vi "Result.Parse STD OUT Text, Create Result Data.vi"(4 "UUTDir":path, 6 "Prefix":string, 7 "Category":string, 8 "Version Name":string, 9 "Error Code":i32, 10 "Task Name":string, 11 "StdOut":string) -> (0 "Error":errorcluster, 1 "SW Ver":T4[](array[typedef]), 3 "Meas":T2[](array[typedef]) {"Status" items=["LOG", "PASS", "FAIL", "ERROR"]}, 5 "Data Files":T1[](array[typedef]))   [LabVIEW 2024]
uses:
  Result XML/TestResult.SW Item.ctl
  Result.Measurement Item.ctl
  Result.Measurement and Attribute Item Status.ctl
  Reports/Report.Result FileDataObject.ctl
  Errors/Error.Error Code List.ctl
  <vilib>/Utility/error.llb/Trim Whitespace One-Sided.vi
  <vilib>/KATE/Files/File Utils.lvlib
  Errors.lvlib
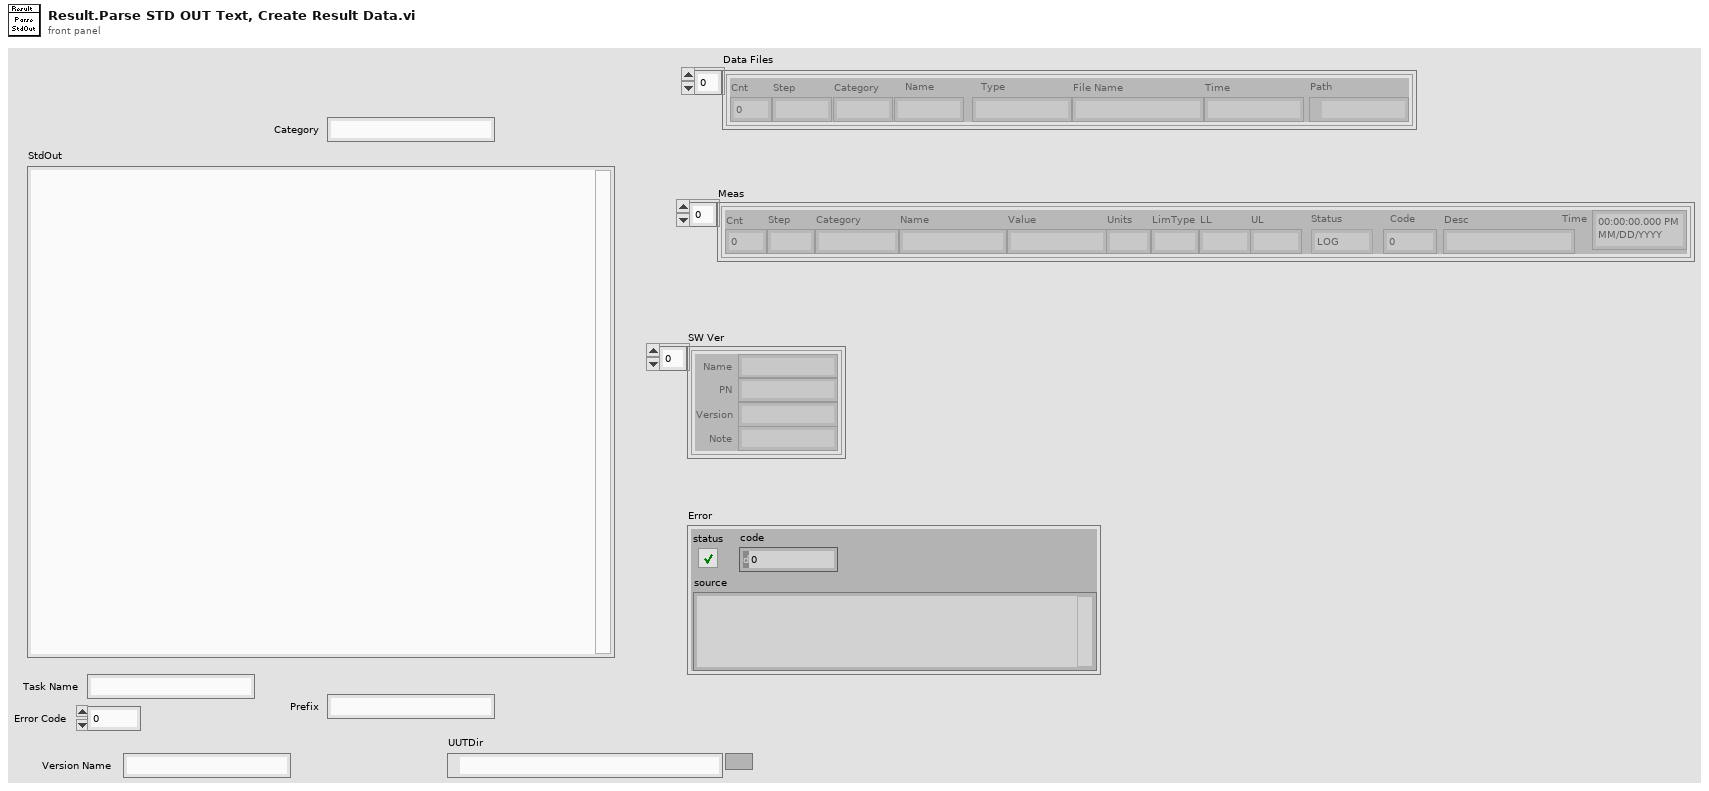
[diagram p1: front panel]
types:
  T1 = typedef "Report.Result FileDataObject.ctl" = cluster{"Cnt":i32, "Step":string, "Category":string, "Name":string, "Type":string, "File Name":string, "Time":string, "Path":path}
  T2 = typedef "Result.Measurement Item.ctl" = cluster{"Cnt":i32, "Step":string, "Category":string, "Name":string, "Value":string, "Units":string, "LimType":string, "LL":string, "UL":string, "Status":T3, "Code":i32, "Desc":string, "Time":timestamp}
  T3 = typedef "Result.Measurement and Attribute Item Status.ctl" = i32
  T4 = typedef "TestResult.SW Item.ctl" = cluster{"Name":string, "PN":string, "Version":string, "Note":string}
  T5 = cluster{"Meas":T2[], "SW Ver":T4[], "Error":errorcluster, "Data Files":T1[]}
  T6 = typedef "EQMF.lvlib/Errors.lvlib/Error.Error Code List.ctl" = i32
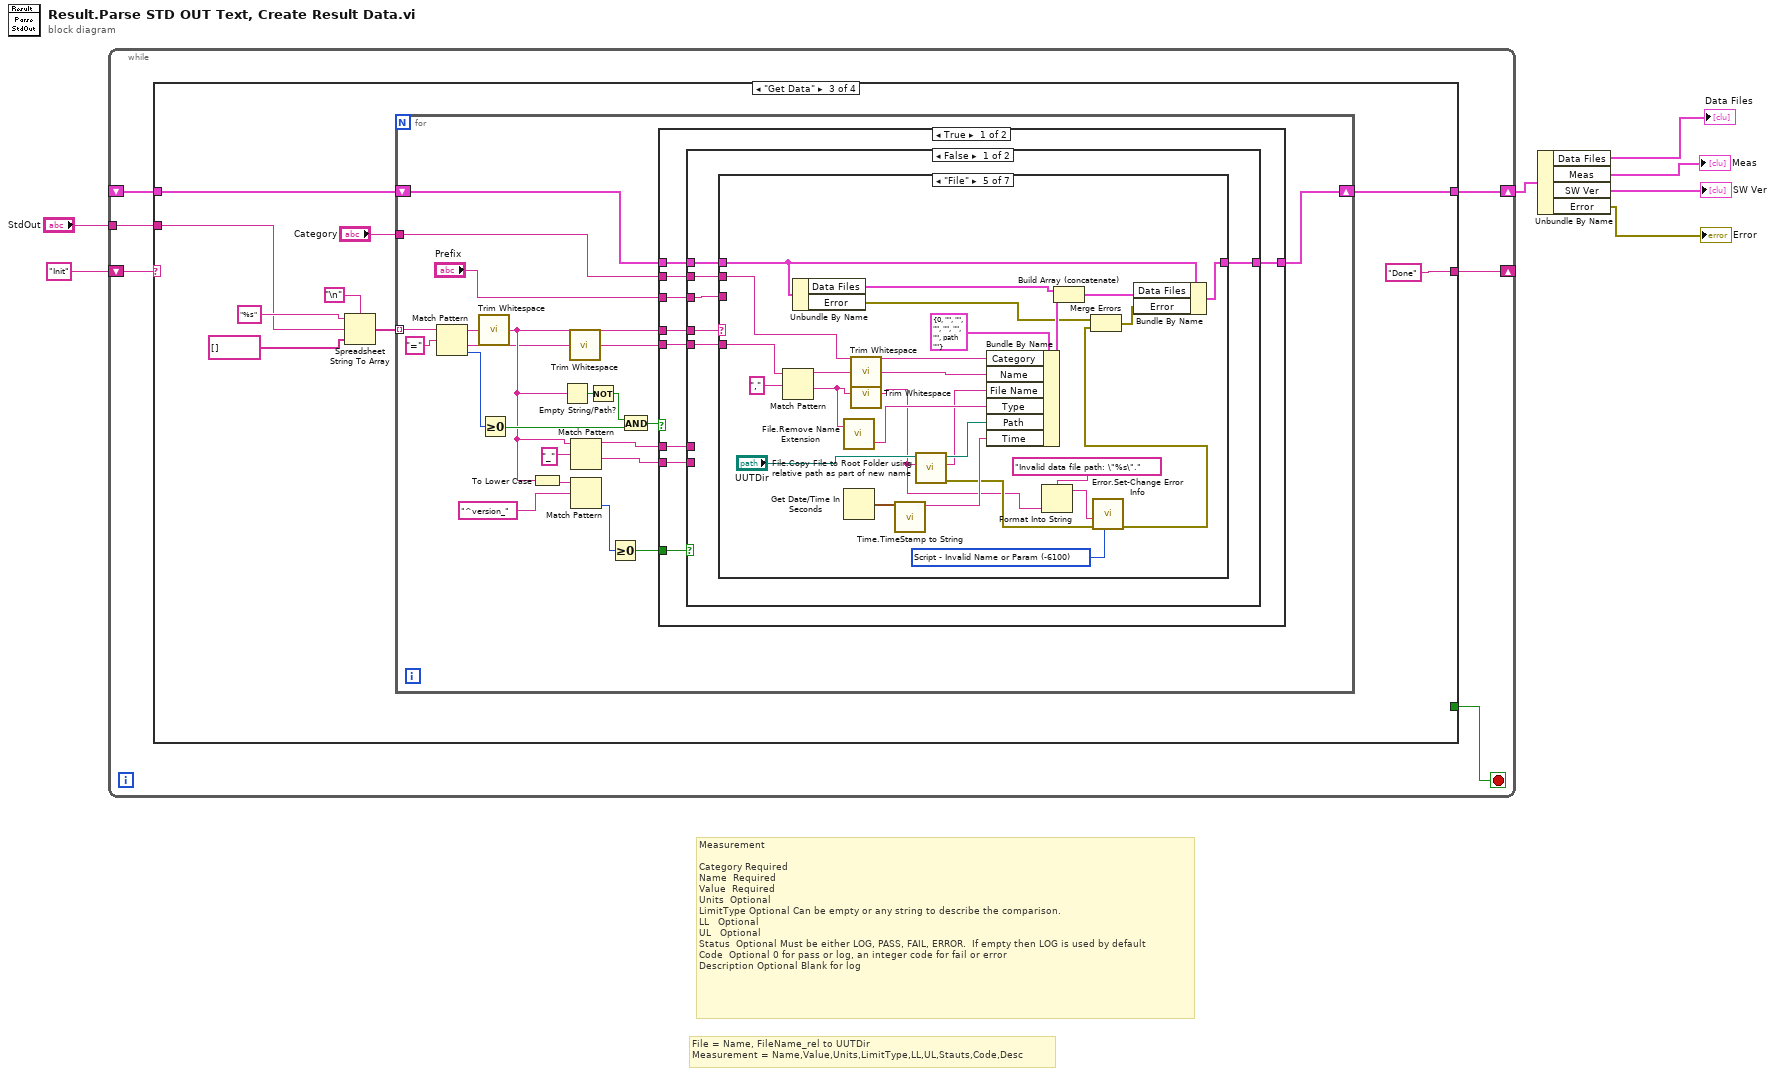
[diagram p0: block diagram]
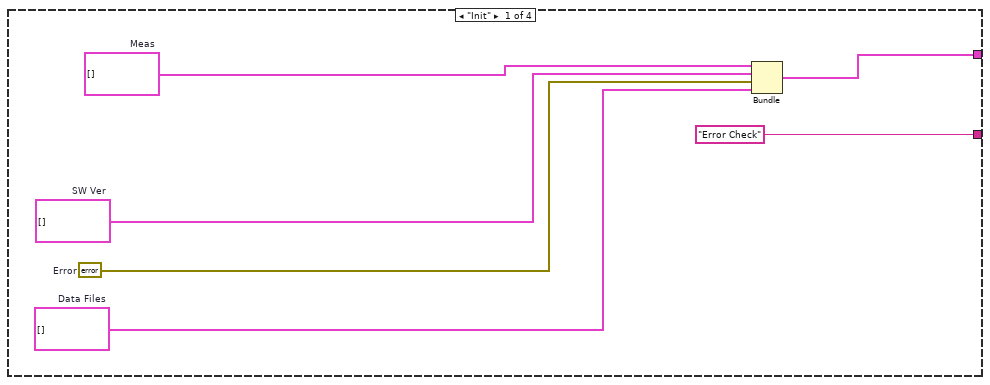
[diagram p2: hidden frame]
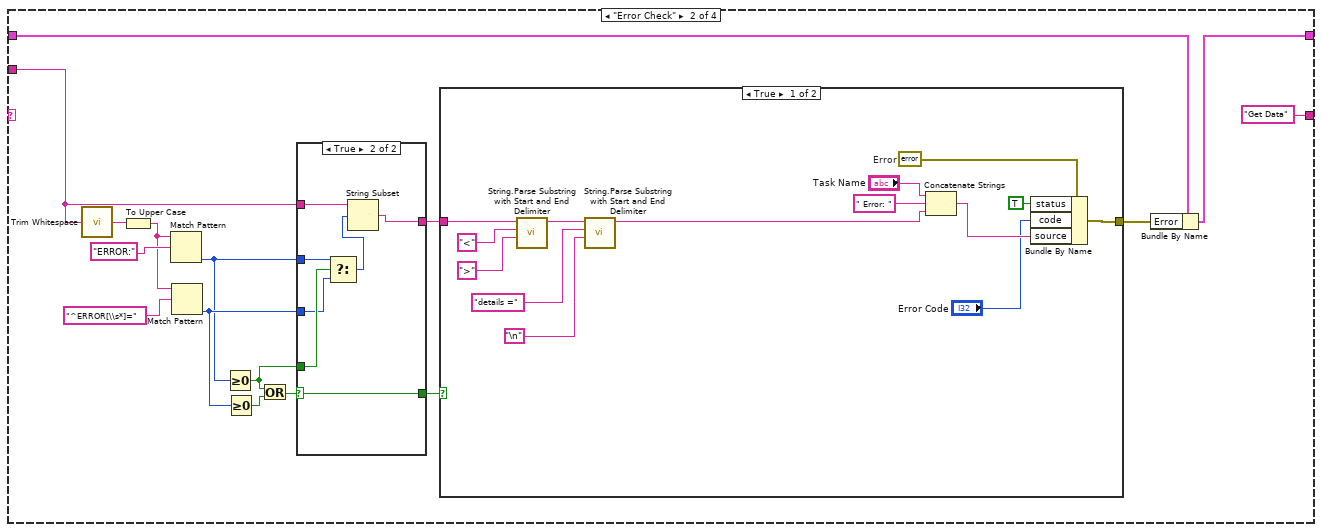
[diagram p3: hidden frame]
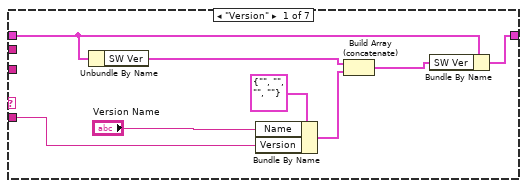
[diagram p6: hidden frame]
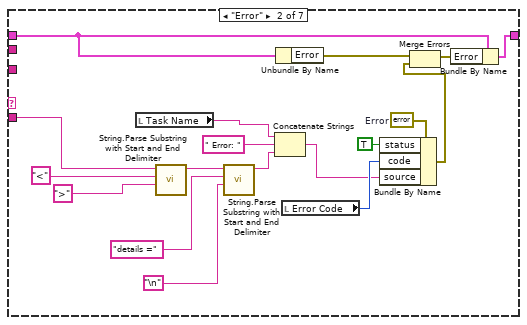
[diagram p7: hidden frame]
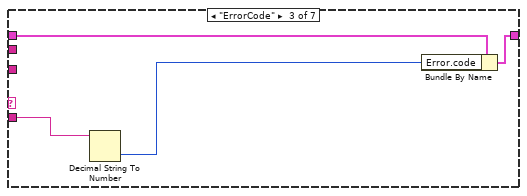
[diagram p8: hidden frame]
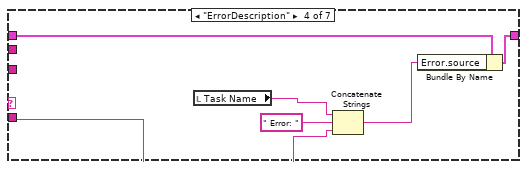
[diagram p9: hidden frame]
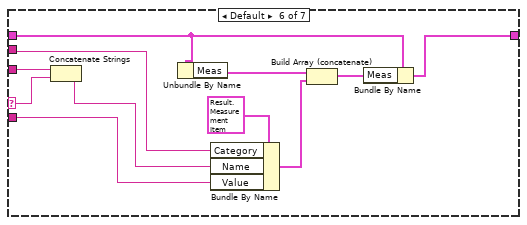
[diagram p10: hidden frame]
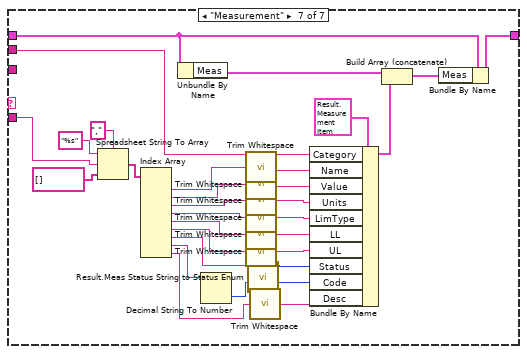
[diagram p11: hidden frame]
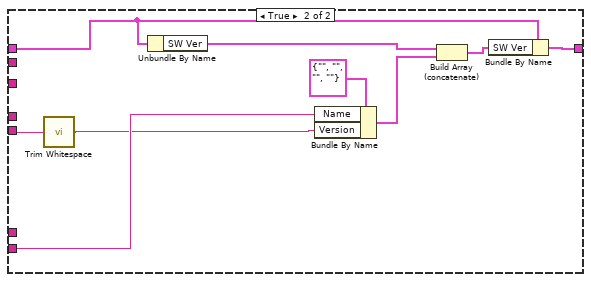
[diagram p12: hidden frame]
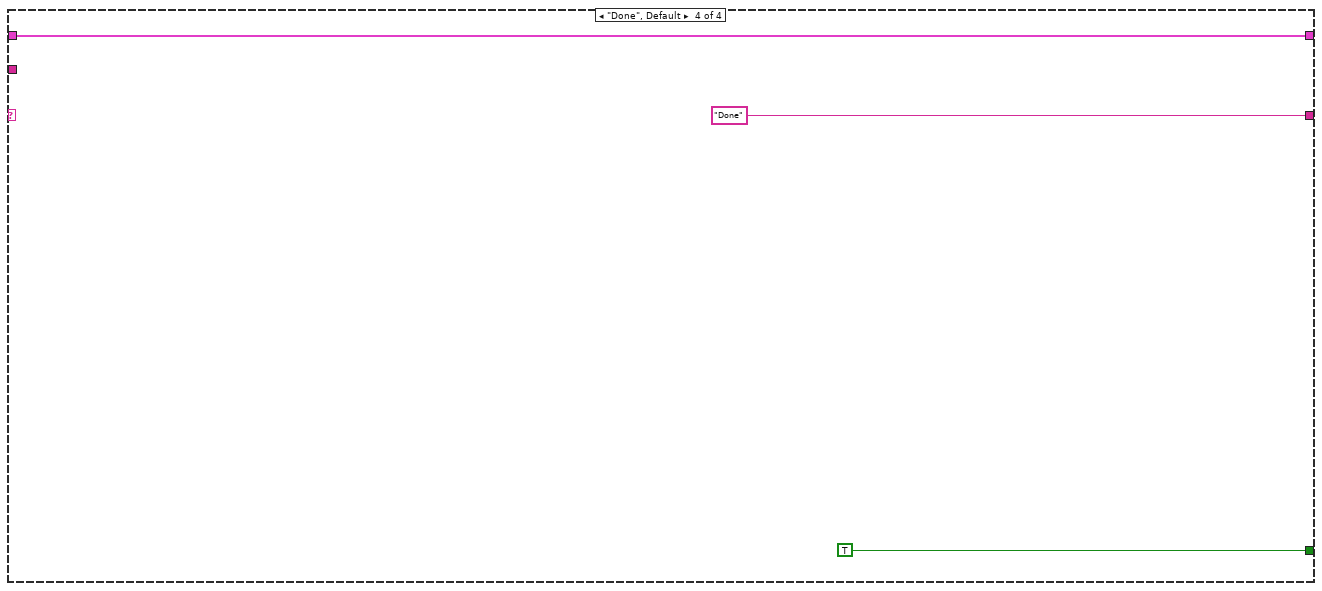
[diagram p14: hidden frame]
diagram:
  # "File = Name, FileName_rel to UUTDir\nMeasurement = Name,Value,Units,LimitType,LL,UL,Stauts,Code,Desc"
  # "Measurement\n\nCategory\tRequired\nName\t\tRequired\nValue\t\tRequired\nUnits\t\tOptional\t\nLimitType\tOptional\tCan be empty or any string to describe the comparison. \nLL \t\tOptional\nUL \t\tOptional\nStatus\t\tOptional\tMust be either LOG, PASS, FAIL, ERROR.  If empty then LOG is used by default\nCode\t\tOptional\t0 for pass or log, an integer code for fail or error\nDescription\tOptional\tBlank for log"
  n1 = while {
    tunnel: "StdOut" -> [w13]
    shift-right: [w9] -> _
    shift-left: "Init" -> [w12]
    shift-right: [w10] -> w5
    shift-left: _ -> [w11]
    stop <- w8 stop-if-true
    n2 = case shown="\"Get Data\"" w12 {
      tunnel: w13 -> [_ w20 w63 _]
      tunnel: w11 -> [_ w34 w60 w217]
      tunnel: [w17 w33 w58 w217] -> w10
      tunnel: ["Error Check" "Get Data" "Done" "Done"] -> w9
      tunnel: [_ _ _ TRUE] -> w8
      frame "Init" {
        w14 = T1[] []  # Data Files
        w15 = errorcluster {"status"=FALSE, "code"=0, "source"=""}  # Error
        w19 = T2[] []  # Meas
        w18 = T4[] []  # SW Ver
        n3 = Bundle("Meas"=w19, "SW Ver"=w18, "Error"=w15, "Data Files"=w14) -> (w17:T5)  [unwired: 1 in]
      }
      frame "Error Check" {
        n4 = call <vilib>:"Trim Whitespace.vi"("string"=w20) -> ("trimmed string"=w21:string)  [unwired: 1 in]
        n5 = To Upper Case(1:w21) -> (0:w29:string)
        n6 = Match Pattern(string=w29, regular expression="ERROR:") -> (offset past match=w25:i32)  [unwired: 1 in, 3 out]
        n7 = Match Pattern(string=w29, regular expression="^ERROR[\\s*]=") -> (offset past match=w26:i32)  [unwired: 1 in, 3 out]
        n8 = Greater Or Equal To 0?(x=w25) -> (x >= 0?=w24:bool)
        n9 = Greater Or Equal To 0?(x=w26) -> (x >= 0?=w28:bool)
        n10 = Or(x=w24, y=w28) -> (x .or. y?=w27:bool)
        n11 = case shown="True" w27 {
          selector: w27 -> [w36 w37]
          tunnel: w26 -> [_ w40]
          tunnel: w25 -> [_ w42]
          tunnel: w20 -> [_ w43]
          tunnel: w24 -> [_ w41]
          tunnel: [_ w38] -> w23
          tunnel: [w36 w37] -> w22
          frame False {
          }
          frame True {
            n12 = Select(t=w42, s=w41, f=w40) -> (s? t:f=w39:i32)
            n13 = String Subset(string=w43, offset (0)=w39) -> (substring=w38:string)  [unwired: 1 in]
          }
        }
        n14 = case shown="True" w22 {
          tunnel: w23 -> [w50 _]
          tunnel: [w51 _] -> w31
          frame True {
            w57 = errorcluster {"status"=FALSE, "code"=0, "source"=""}  # Error
            n15 = call "String.Parse Substring with Start and End Delimiter.vi"("Delimiter2"=">", "Delimiter1"="<", "String In"=w50) -> ("String Out"=w47:string)  [unwired: 7 in, 1 out]
            n16 = call "String.Parse Substring with Start and End Delimiter.vi"("Delimiter2"="\n", "Delimiter1"="details =", "String In"=w47) -> ("String Out"=w44:string)  [unwired: 7 in, 1 out]
            n17 = Concatenate Strings("Task Name", " Error: ", w44) -> (w53:string)
            n18 = Bundle By Name(cluster=w57, "status"=TRUE, "code"="Error Code", "source"=w53) -> (w51:errorcluster)
          }
          frame False {
          }
        }
        n19 = Bundle By Name(cluster=w34, "Error"=w31) -> (w33:T5)
      }
      frame "Get Data" {
        n20 = Spreadsheet String To Array(delimiter (Tab)="\n", format string="%s" ("spreadsheet string"), spreadsheet string=w63, array type (2D Dbl)=string[] []) -> (array=w61:string[])
        n21 = for {
          tunnel: w61 -> [w88] mode=indexing
          shift-right: [w85] -> w58
          shift-left: w60 -> [w86]
          tunnel: "Category" -> [w78]
          n22 = Match Pattern(string=w88, regular expression="=") -> (before substring=w84:string, after substring=w68:string, offset past match=w83:i32)  [unwired: 1 in, 1 out]
          n23 = call <vilib>:"Trim Whitespace.vi"("string"=w84) -> ("trimmed string"=w69:string)  [unwired: 1 in]
          n24 = Greater Or Equal To 0?(x=w83) -> (x >= 0?=w80:bool)
          n25 = To Lower Case(string=w69) -> (all lower case string=w73:string)
          n26 = Empty String/Path?(string/path=w69) -> (empty?=w82:bool)
          n27 = call <vilib>:"Trim Whitespace.vi"("string"=w68) -> ("trimmed string"=w67:string)  [unwired: 1 in]
          n28 = Match Pattern(string=w69, regular expression="_") -> (before substring=w72:string, after substring=w71:string)  [unwired: 1 in, 2 out]
          n29 = Match Pattern(string=w73, regular expression="^version_") -> (offset past match=w76:i32)  [unwired: 1 in, 3 out]
          n30 = Not(x=w82) -> (.not. x?=w81:bool)
          n31 = Greater Or Equal To 0?(x=w76) -> (x >= 0?=w75:bool)
          n32 = And(x=w81, y=w80) -> (x .and. y?=w79:bool)
          n33 = case shown="True" w79 {
            tunnel: w86 -> [w95 w216]
            tunnel: [w94 w216] -> w85
            tunnel: w67 -> [w97 _]
            tunnel: w69 -> [w93 _]
            tunnel: w78 -> [w96 _]
            tunnel: "Prefix" -> [w92 _]
            tunnel: w72 -> [w89 _]
            tunnel: w71 -> [w90 _]
            tunnel: w75 -> [w91 _]
            frame True {
              n34 = case shown="False" w91 {
                tunnel: w97 -> [w103 w208]
                tunnel: w96 -> [w102 _]
                tunnel: w95 -> [w101 w210]
                tunnel: [w100 w211] -> w94
                tunnel: w93 -> [w99 _]
                tunnel: w92 -> [w98 _]
                tunnel: w90 -> [_ w209]
                tunnel: w89 -> [_ _]
                frame False {
                  n35 = case shown="\"File\"" w99 {
                    selector: w99 -> [_ _ _ _ _ w171 _]
                    tunnel: w103 -> [w104 w112 w130 w135 w152 w176 w196]
                    tunnel: w102 -> [_ _ _ _ w159 w172 w204]
                    tunnel: w101 -> [w110 w128 w133 w139 w148 w175 w206]
                    tunnel: [w109 w129 w132 w138 w165 w174 w205] -> w100
                    tunnel: w98 -> [_ _ _ _ _ w173 _]
                    frame "Version" {
                      n36 = Unbundle By Name(w110) -> ("SW Ver"=w107:T4[])
                      n37 = Bundle By Name(cluster=T4 {"Name"="", "PN"="", "Version"="", "Note"=""} ("SW_Item"), "Name"="Version Name", "Version"=w104) -> (w106:T4)
                      n38 = Build Array (concatenate)(w107, w106) -> (w108:T4[])
                      n39 = Bundle By Name(cluster=w110, "SW Ver"=w108) -> (w109:T5)
                    }
                    frame "Error" {
                      w115 = errorcluster {"status"=FALSE, "code"=0, "source"=""}  # Error
                      n40 = local read "Task Name"() -> (w124:string)
                      n41 = call "String.Parse Substring with Start and End Delimiter.vi"("Delimiter2"=">", "Delimiter1"="<", "String In"=w112) -> ("String Out"=w122:string)  [unwired: 7 in, 1 out]
                      n42 = call "String.Parse Substring with Start and End Delimiter.vi"("Delimiter2"="\n", "Delimiter1"="details =", "String In"=w122) -> ("String Out"=w123:string)  [unwired: 7 in, 1 out]
                      n43 = Concatenate Strings(w124, " Error: ", w123) -> (w121:string)
                      n44 = Unbundle By Name(w128) -> ("Error"=w126:errorcluster)
                      n45 = local read "Error Code"() -> (w125:i32)
                      n46 = Bundle By Name(cluster=w115, "status"=TRUE, "code"=w125, "source"=w121) -> (w113:errorcluster)
                      n47 = Merge Errors(w126, w113) -> (w127:errorcluster)
                      n48 = Bundle By Name(cluster=w128, "Error"=w127) -> (w129:T5)
                    }
                    frame "ErrorCode" {
                      n49 = Decimal String To Number(string=w130) -> (number=w131:i32)  [unwired: 2 in, 1 out]
                      n50 = Bundle By Name(cluster=w133, "Error.code"=w131) -> (w132:T5)
                    }
                    frame "ErrorDescription" {
                      n51 = local read "Task Name"() -> (w137:string)
                      n52 = Concatenate Strings(w137, " Error: ", w135) -> (w134:string)
                      n53 = Bundle By Name(cluster=w139, "Error.source"=w134) -> (w138:T5)
                    }
                    frame "File" {
                      w144 = T6 -6100 items=["No Error"=0, "Abort"=-2, "Misc"=-5000, "Fixture Error"=-5100, "File IO - General"=-5200, "FIle IO - Config Error"=-5201, "Instrument - General"=-5300, "Instrument - Serial Com"=-5301, "Instrument - Camera"=-5302, "Instrument - PS"=-5303, "Instrument - Oscilloscope"=-5304, "Instrument - Function Gen"=-5305, "Instrument - Load"=-5306, "Instrument - Meter"=-5307, "Instrument - Power Control"=-5308, "Instrument - Motion"=-5309, "Instrument - RF"=-5310, "System Exe"=-5400, "Image Processing"=-5500, "Communication"=-5600, "Script - Syntax Error"=-6000, "Script - Invalid Name or Param"=-6100, "Script - Timeout"=-6200, "Invalid Data"=-6300, "FW Update Error"=-6500] ("Std Code")
                      n54 = Match Pattern(string=w152, regular expression=",") -> (before substring=w157:string, after substring=w155:string)  [unwired: 1 in, 2 out]
                      n55 = Unbundle By Name(w148) -> ("Data Files"=w163:T1[], "Error"=w146:errorcluster)
                      n56 = call <vilib>:"File.Remove Name Extension.vi"("File Name"=w155) -> ("Ext"=w156:string)  [unwired: 1 in, 1 out]
                      n57 = Get Date/Time In Seconds() -> (seconds since 1Jan1904=w154:timestamp)
                      n58 = call <vilib>:"Trim Whitespace.vi"("string"=w157) -> ("trimmed string"=w158:string)  [unwired: 1 in]
                      n59 = call <vilib>:"Trim Whitespace.vi"("string"=w155) -> ("trimmed string"=w141:string)  [unwired: 1 in]
                      n60 = call "Time.TimeStamp to String.vi"("Time Stamp in"=w154) -> ("Time String Out"=w153:string)  [unwired: 10 in]
                      n61 = call "File.Copy File to Root Folder using relative path as part of new name.vi"("Relative Path"=w141, "Root Path"="UUTDir") -> ("error out"=w145:errorcluster, "New File Name"=w149:string, "Adjusted Path"=w150:path)  [unwired: 6 in, 1 out]
                      n62 = Bundle By Name(cluster=T1 {"Cnt"=0, "Step"="", "Category"="", "Name"="", "Type"="", "File Name"="", "Time"="", "Path"=path ""} ("FileData Object"), "Category"=w159, "Name"=w158, "File Name"=w149, "Type"=w156, "Path"=w150, "Time"=w153) -> (w162:T1)
                      n63 = Format Into String(format string="Invalid data file path: \"%s\".", w141) -> (resulting string=w142:string)  [unwired: 2 in, 1 out]
                      n64 = Build Array (concatenate)(w163, w162) -> (w164:T1[])
                      n65 = call "Error.Set-Change Error Info.vi"("Std Code"=w144, "error in"=w145, "Description"=w142) -> ("error out"=w140:errorcluster)  [unwired: 8 in]
                      n66 = Merge Errors(w146, w140) -> (w147:errorcluster)
                      n67 = Bundle By Name(cluster=w148, "Data Files"=w164, "Error"=w147) -> (w165:T5)
                    }
                    frame Default {
                      n68 = Concatenate Strings(w173, w171) -> (w170:string)
                      n69 = Unbundle By Name(w175) -> ("Meas"=w168:T2[])
                      n70 = Bundle By Name(cluster=T2 {"Cnt"=0, "Step"="", "Category"="", "Name"="", "Value"="", "Units"="", "LimType"="", "LL"="", "UL"="", "Status"=0, "Code"=0, "Desc"="", "Time"=timestamp(0 s since 1904-01-01)} ("Meas"), "Category"=w172, "Name"=w170, "Value"=w176) -> (w167:T2)
                      n71 = Build Array (concatenate)(w168, w167) -> (w166:T2[])
                      n72 = Bundle By Name(cluster=w175, "Meas"=w166) -> (w174:T5)
                    }
                    frame "Measurement" {
                      n73 = Spreadsheet String To Array(delimiter (Tab)="," ("spreadsheet string"), format string="%s" ("spreadsheet string"), spreadsheet string=w196, array type (2D Dbl)=string[] []) -> (array=w195:string[])
                      n74 = Index Array(array=w195) -> (element #1=w194:string, element #2=w193:string, element #3=w190:string, element #4=w189:string, element #5=w188:string, element #6=w187:string, element #7=w180:string, element #8=w179:string, element #9=w177:string)  [unwired: 9 in]
                      n75 = Unbundle By Name(w206) -> ("Meas"=w202:T2[])
                      n76 = Decimal String To Number(string=w179) -> (number=w178:i32)  [unwired: 2 in, 1 out]
                      n77 = call <vilib>:"Trim Whitespace.vi"("string"=w194) -> ("trimmed string"=w192:string)  [unwired: 1 in]
                      n78 = call <vilib>:"Trim Whitespace.vi"("string"=w193) -> ("trimmed string"=w191:string)  [unwired: 1 in]
                      n79 = call <vilib>:"Trim Whitespace.vi"("string"=w190) -> ("trimmed string"=w186:string)  [unwired: 1 in]
                      n80 = call <vilib>:"Trim Whitespace.vi"("string"=w189) -> ("trimmed string"=w185:string)  [unwired: 1 in]
                      n81 = call <vilib>:"Trim Whitespace.vi"("string"=w188) -> ("trimmed string"=w182:string)  [unwired: 1 in]
                      n82 = call <vilib>:"Trim Whitespace.vi"("string"=w187) -> ("trimmed string"=w184:string)  [unwired: 1 in]
                      n83 = call "Result.Meas Status String to Status Enum.vi"("Status Str"=w180) -> ("Status"=w181:T3)  [unwired: 10 in]
                      n84 = call <vilib>:"Trim Whitespace.vi"("string"=w177) -> ("trimmed string"=w183:string)  [unwired: 1 in]
                      n85 = Bundle By Name(cluster=T2 {"Cnt"=0, "Step"="", "Category"="", "Name"="", "Value"="", "Units"="", "LimType"="", "LL"="", "UL"="", "Status"=0, "Code"=0, "Desc"="", "Time"=timestamp(0 s since 1904-01-01)} ("Meas"), "Category"=w204, "Name"=w192, "Value"=w191, "Units"=w186, "LimType"=w185, "LL"=w182, "UL"=w184, "Status"=w181, "Code"=w178, "Desc"=w183) -> (w201:T2)
                      n86 = Build Array (concatenate)(w202, w201) -> (w200:T2[])
                      n87 = Bundle By Name(cluster=w206, "Meas"=w200) -> (w205:T5)
                    }
                  }
                }
                frame True {
                  n88 = call <vilib>:"Trim Whitespace.vi"("string"=w208) -> ("trimmed string"=w207:string)  [unwired: 1 in]
                  n89 = Unbundle By Name(w210) -> ("SW Ver"=w213:T4[])
                  n90 = Bundle By Name(cluster=T4 {"Name"="", "PN"="", "Version"="", "Note"=""} ("SW_Item"), "Name"=w209, "Version"=w207) -> (w212:T4)
                  n91 = Build Array (concatenate)(w213, w212) -> (w214:T4[])
                  n92 = Bundle By Name(cluster=w210, "SW Ver"=w214) -> (w211:T5)
                }
              }
            }
            frame False {
            }
          }
        }
      }
      frame "Done", Default {
      }
    }
  }
  n93 = Unbundle By Name(w5) -> ("Data Files"=→"Data Files":T1[], "Meas"=→"Meas":T2[], "SW Ver"=→"SW Ver":T4[], "Error"=→"Error":errorcluster)
